vi "EOL CAN_Send_Single_Message.vi"(4 "Retries":i32=2, 6 "Msg Wait Time":u32=100, 7 "Rx Arbitration Id":u32=402522244 format="%.0x", 8 "Error in":errorcluster, 9 "Tx CAN frame":T1={"timestamp"=timestamp(0 s since 1904-01-01), "payload"=[2, 39, 3, 85, 85, 85, 85, 85], "identifier"=402391172, "type"=0, "extended?"=TRUE, "echo?"=FALSE} {"payload" format="%x"; "timestamp" format="%<%.7X\n%x>T"; "type" items=["CAN Data"=0, "CAN Remote"=1, "CAN Bus Error"=2, "CAN 2.0 Data"=8, "CAN FD Data"=16, "CAN FD+BRS Data"=24, "J1939 Data"=192, "Delay"=224, "Log Trigger"=225, "Start Trigger"=226]; "identifier" format="%x"}, 10 "Read Session in":refnum<k21>, 11 "Write Session in":refnum<k21>) -> (0 "Error out":errorcluster, 1 "Rx Message":u8[](array[numeric]) format="%02x", 2 "spreadsheet string":string, 3 "Response Good?":bool, 5 "TxRx Data":string[][](array[string]))   [LabVIEW 2018]
uses:
  <vilib>/xnet/xnet.llb/XNET Frame CAN.ctl
  <vilib>/xnet/xnet.llb/XNET Frame Type CAN.ctl
  <vilib>/xnet/xnet.llb/XNET Write (Frame CAN).vi
  <vilib>/xnet/xnet.llb/XNET Read (Frame CAN).vi
panel:
  # "17FC0084"
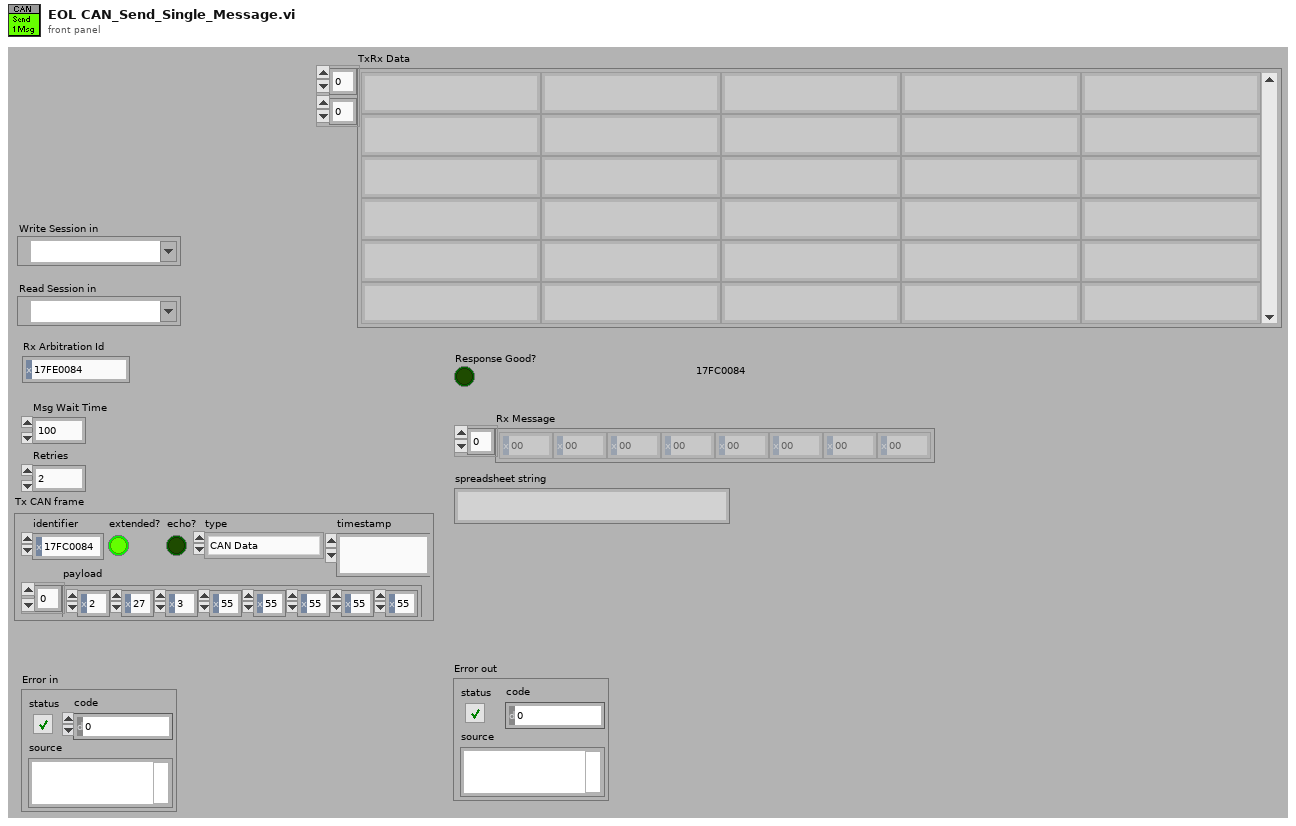
[diagram p1: front panel]
types:
  T1 = typedef "XNET Frame CAN.ctl" = cluster{"timestamp":timestamp, "payload":u8[], "identifier":u32, "type":T2, "extended?":bool, "echo?":bool}
  T2 = typedef "XNET Frame Type CAN.ctl" = u8
  T3 = cluster{"Read Session in":refnum<k21>, "Write Session in":refnum<k21>, "Tx CAN frame":T1, "Rx Arbitration Id":u32, "Retry Counter":i32, "Rx Msg":u8[], "Response Good?":bool, "TxRx Data":string[][], "Message Start Timer":u32, "Message Wait Timer":i32, "Error in":errorcluster}
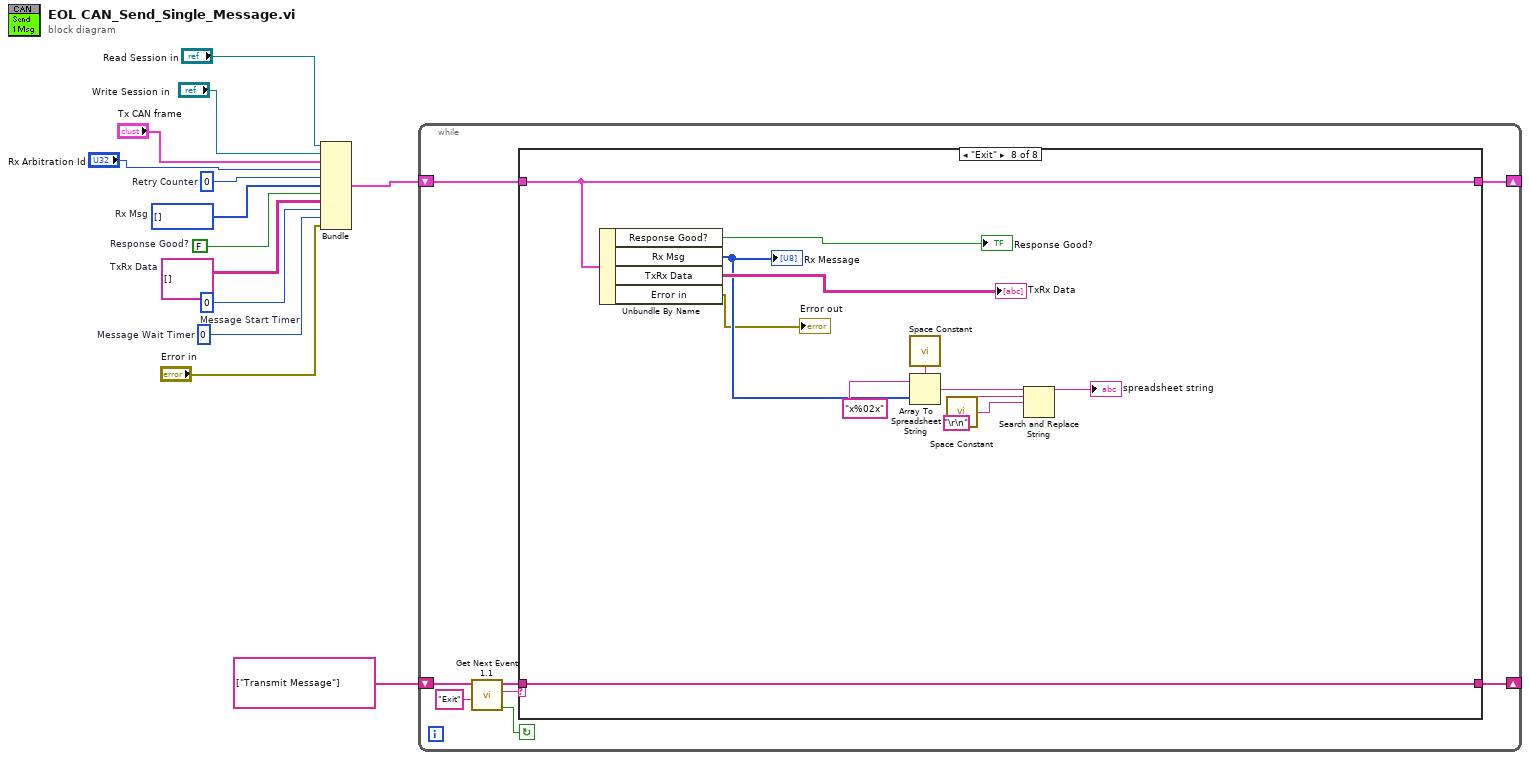
[diagram p0: block diagram]
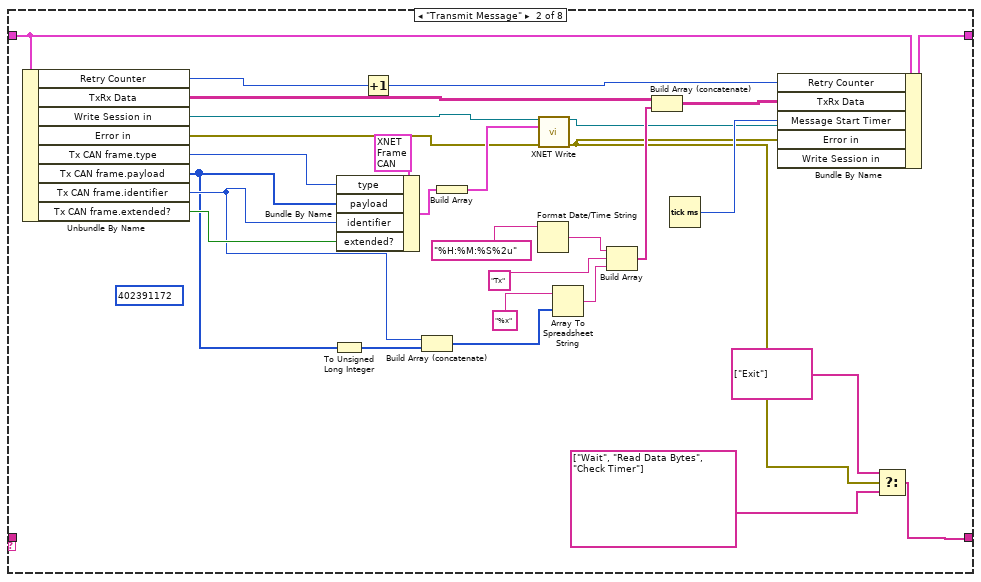
[diagram p3: hidden frame]
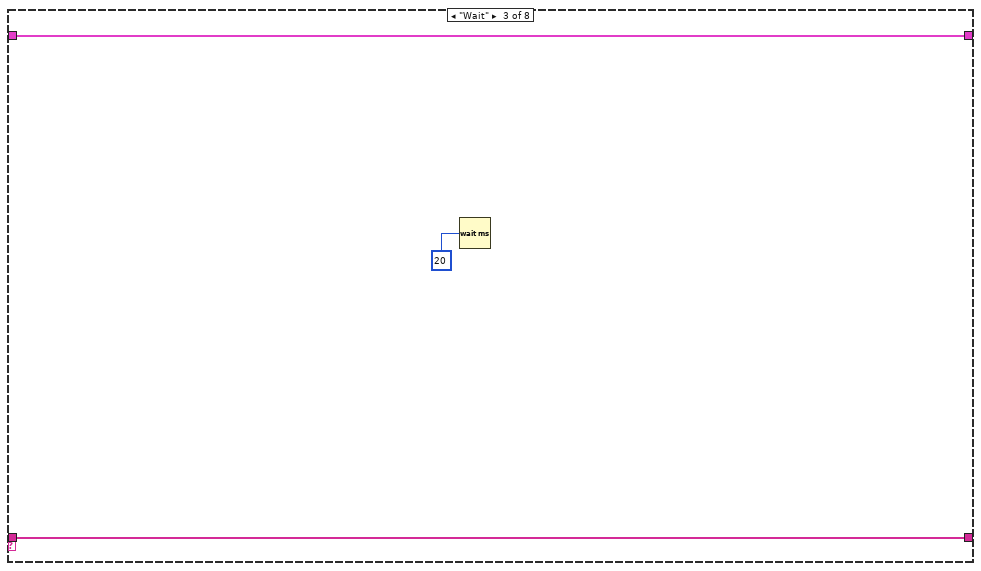
[diagram p4: hidden frame]
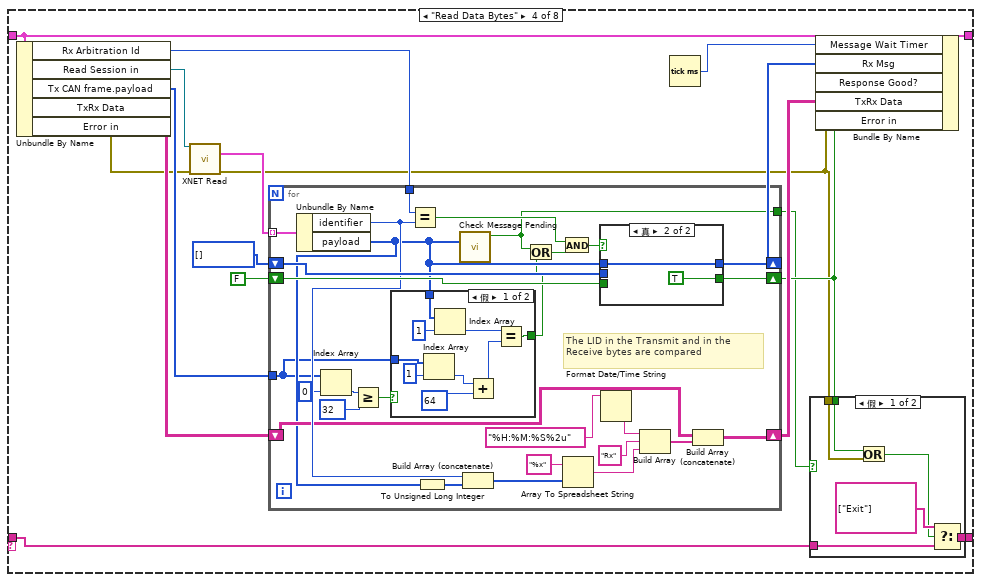
[diagram p5: hidden frame]
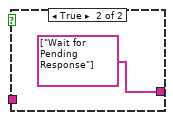
[diagram p6: hidden frame]
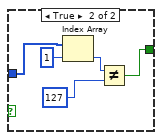
[diagram p7: hidden frame]
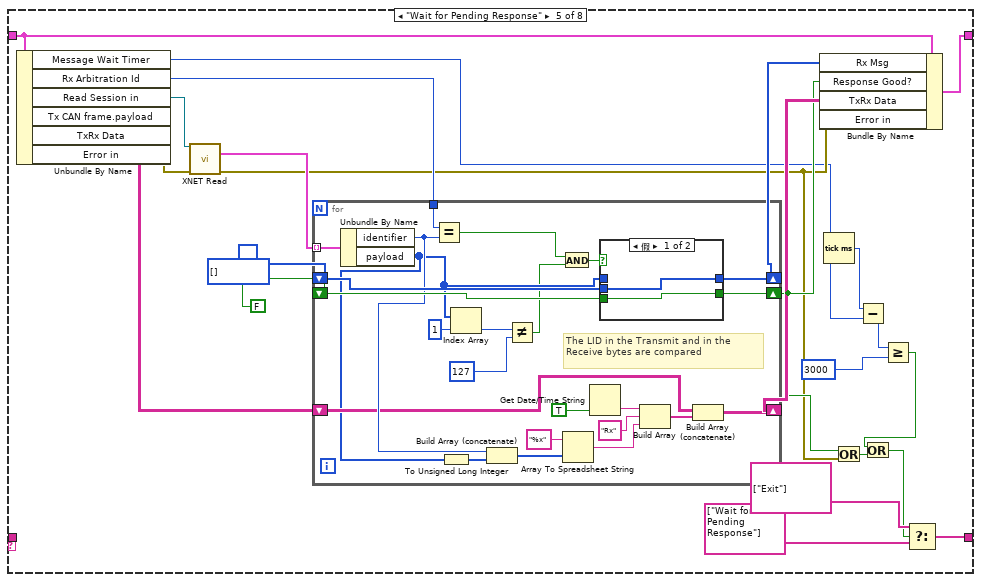
[diagram p9: hidden frame]
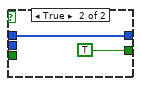
[diagram p10: hidden frame]
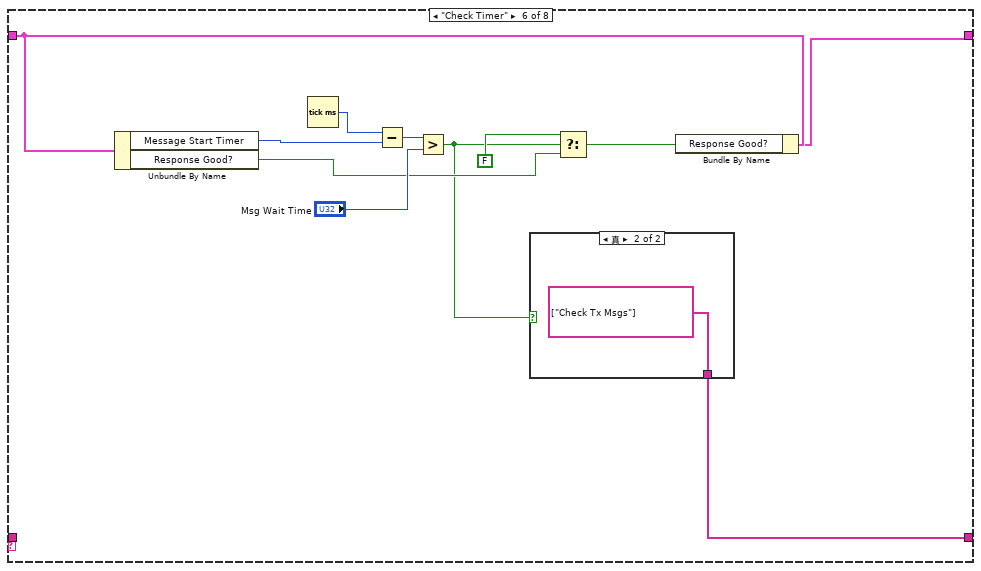
[diagram p11: hidden frame]
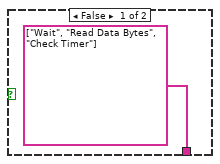
[diagram p12: hidden frame]
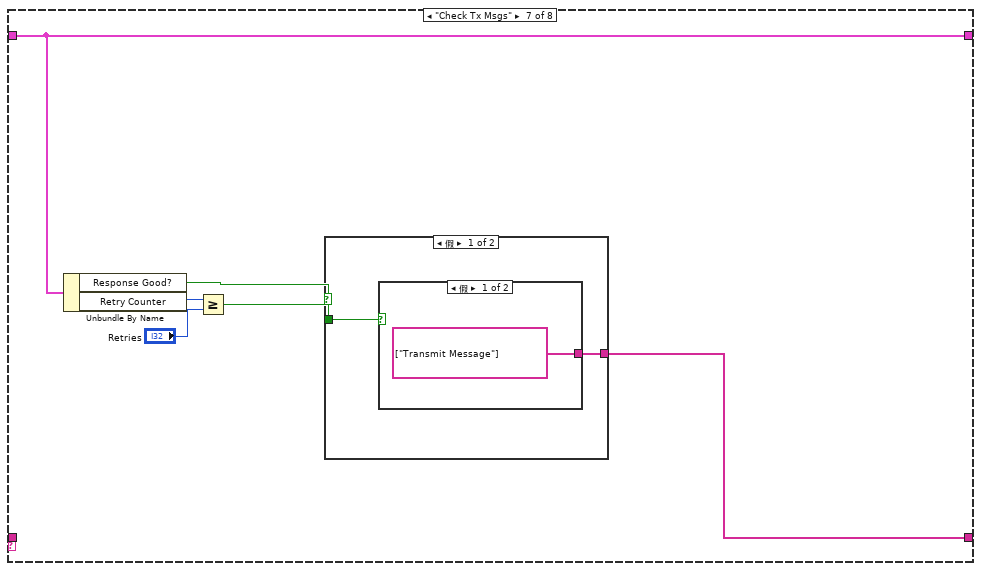
[diagram p13: hidden frame]
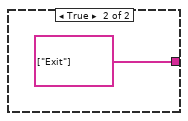
[diagram p14: hidden frame]
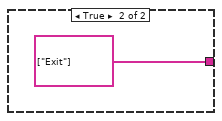
[diagram p15: hidden frame]
diagram:
  w1 = 0  # Message Wait Timer
  w7 = u32 0  # Message Start Timer
  w8 = string[][] []  # TxRx Data
  w9 = FALSE  # Response Good?
  w10 = u8[] []  # Rx Msg
  w12 = 0  # Retry Counter
  n1 = Bundle("Read Session in"="Read Session in", "Write Session in"="Write Session in", "Tx CAN frame"="Tx CAN frame", "Rx Arbitration Id"="Rx Arbitration Id", "Retry Counter"=w12, "Rx Msg"=w10, "Response Good?"=w9, "TxRx Data"=w8, "Message Start Timer"=w7, "Message Wait Timer"=w1, "Error in"="Error in") -> (w11:T3)  [unwired: 1 in]
  n2 = while {
    shift-right: [w18] -> _
    shift-left: string[] ["Transmit Message"] ("event queue out") -> [w17]
    shift-right: [w15] -> _
    shift-left: w11 -> [w16]
    stop <- w21 continue-if-true
    n3 = call "Get Next Event 1.1.vi"("Exit Event"="Exit", "event queue in"=w17) -> ("Condition (Exit:F)"=w21:bool, "next event"=w20:string, "event queue out"=w19:string[])  [unwired: 6 in, 1 out]
    n4 = case shown="\"Exit\"" w20 {
      tunnel: w19 -> [w23 _ w53 w68 _ _ _ w213]
      tunnel: [w23 w32 w53 w67 w145 w178 w193 w213] -> w18
      tunnel: w16 -> [w22 w51 w54 w73 w149 w180 w191 w212]
      tunnel: [w22 w49 w54 w72 w148 w179 w191 w212] -> w15
      frame "Error", Default {
      }
      frame "Transmit Message" {
        (unwired) u32 402391172 ("Tx Arbitration Id")
        n5 = Unbundle By Name(w51) -> ("Retry Counter"=w52:i32, "TxRx Data"=w46:string[][], "Write Session in"=w27:refnum<k21>, "Error in"=w26:errorcluster, "Tx CAN frame.type"=w33:T2, "Tx CAN frame.payload"=w34:u8[], "Tx CAN frame.identifier"=w35:u32, "Tx CAN frame.extended?"=w36:bool)
        n6 = To Unsigned Long Integer(number=w34) -> (unsigned 32bit integer=w45:u32[])
        n7 = Bundle By Name(cluster=T1 {"timestamp"=timestamp(0 s since 1904-01-01), "payload"=[2, 39, 3, 85, 85, 85, 85, 85], "identifier"=402391172, "type"=8, "extended?"=TRUE, "echo?"=FALSE} ("CAN frame"), "type"=w33, "payload"=w34, "identifier"=w35, "extended?"=w36) -> (w39:T1)
        n8 = Increment(x=w52) -> (x+1=w50:i32)
        n9 = Build Array (concatenate)(w35, w45) -> (w41:u32[])
        n10 = Build Array(w39) -> (w37:T1[])
        n11 = Format Date/Time String(time format string (%c)="%H:%M:%S%2u" ("时间格式字符串(%c)")) -> (date/time string=w25:string)  [unwired: 2 in]
        n12 = call-poly <vilib>:"XNET Write.vi"("session in"=w27, "data"=w37, "error in (no error)"=w26) -> ("session out"=w28:refnum<k21>, "error out"=w29:errorcluster)  [unwired: 11 in]
        n13 = Array To Spreadsheet String(array=w41, 3:"%x" ("format string")) -> (spreadsheet string=w43:string)  [unwired: 1 in]
        n14 = Build Array(w25, "Tx" ("format string"), w43) -> (w44:string[])
        n15 = Build Array (concatenate)(w46, w44) -> (w47:string[][])
        n16 = Tick Count (ms)() -> (millisecond timer value=w48:u32)
        n17 = Bundle By Name(cluster=w51, "Retry Counter"=w50, "TxRx Data"=w47, "Message Start Timer"=w48, "Error in"=w29, "Write Session in"=w28) -> (w49:T3)
        n18 = Select(t=string[] ["Exit"], s=w29, f=string[] ["Wait", "Read Data Bytes", "Check Timer"] ("event queue out")) -> (s? t:f=w32:string[])
      }
      frame "Wait" {
        n19 = Wait (ms)(milliseconds to wait=u32 20) -> ()  [unwired: 1 out]
      }
      frame "Read Data Bytes" {
        n20 = Unbundle By Name(w73) -> ("Rx Arbitration Id"=w60:u32, "Read Session in"=w70:refnum<k21>, "Tx CAN frame.payload"=w69:u8[], "TxRx Data"=w66:string[][], "Error in"=w64:errorcluster)
        n21 = call-poly <vilib>:"XNET Read.vi"("session in"=w70, "error in (no error)"=w64) -> ("data"=w61:T1[], "error out"=w58:errorcluster)  [unwired: 10 in, 2 out]
        n22 = for {
          tunnel: w61 -> [w108] mode=indexing
          shift-right: [w107] -> w71
          shift-left: u8[] [] ("Data Array") -> [w106]
          shift-right: [w105] -> w59
          shift-left: FALSE -> [w104]
          tunnel: w69 -> [w86]
          shift-right: [w94] -> w65
          shift-left: w66 -> [w95]
          tunnel: w60 -> [w92]
          tunnel: [w88] -> w57
          # "The LID in the Transmit and in the\nReceive bytes are compared"
          n23 = Unbundle By Name(w108) -> ("identifier"=w100:u32, "payload"=w91:u8[])
          n24 = Index Array(array=w86, index=0) -> (element=w85:u8)
          n25 = Greater Or Equal?(x=w85, y=u8 32) -> (x >= y?=w83:bool)
          n26 = case shown="假" w83 {
            tunnel: w91 -> [w114 _]
            tunnel: [w113 w119] -> w90
            tunnel: w86 -> [w112 w118]
            frame False {
              n27 = Index Array(array=w112, index=1) -> (element=w111:u8)
              n28 = Index Array(array=w114, index=1) -> (element=w117:u8)
              n29 = Add(x=w111, y=u8 64 ("Numeric")) -> (x+y=w116:u8)
              n30 = Equal?(x=w117, y=w116) -> (x = y?=w113:bool)
            }
            frame True {
              n31 = Index Array(array=w118, index=1) -> (element=w120:u8)
              n32 = Not Equal?(x=w120, y=u8 127 ("Numeric")) -> (x != y?=w119:bool)
            }
          }
          n33 = Equal?(x=w92, y=w100) -> (x = y?=w102:bool)
          n34 = To Unsigned Long Integer(number=w91) -> (unsigned 32bit integer=w101:u32[])
          n35 = call "Check Message Pending.vi"("Data Array"=w91) -> ("x .and. y?"=w88:bool)  [unwired: 10 in]
          n36 = Build Array (concatenate)(w100, w101) -> (w93:u32[])
          n37 = Or(x=w88, y=w90) -> (x .or. y?=w89:bool)
          n38 = And(x=w102, y=w89) -> (x .and. y?=w103:bool)
          n39 = Array To Spreadsheet String(array=w93, 3:"%x" ("format string")) -> (spreadsheet string=w97:string)  [unwired: 1 in]
          n40 = case shown="真" w103 {
            tunnel: w91 -> [_ w125]
            tunnel: [w123 w125] -> w107
            tunnel: w106 -> [w123 _]
            tunnel: [w124 TRUE] -> w105
            tunnel: w104 -> [w124 _]
            frame False {
            }
            frame True {
            }
          }
          n41 = Format Date/Time String(time format string (%c)="%H:%M:%S%2u" ("时间格式字符串(%c)")) -> (date/time string=w82:string)  [unwired: 2 in]
          n42 = Build Array(w82, "Rx" ("format string"), w97) -> (w96:string[])
          n43 = Build Array (concatenate)(w95, w96) -> (w94:string[][])
        }
        n44 = Tick Count (ms)() -> (millisecond timer value=w56:u32)
        n45 = case shown="假" w57 {
          tunnel: w68 -> [w79 _]
          tunnel: [w78 string[] ["Wait for Pending Response"] ("t")] -> w67
          tunnel: w59 -> [w76 _]
          tunnel: w58 -> [w74 _]
          frame False {
            n46 = Or(x=w76, y=w74) -> (x .or. y?=w75:bool)
            n47 = Select(t=string[] ["Exit"], s=w75, f=w79) -> (s? t:f=w78:string[])
          }
          frame True {
          }
        }
        n48 = Bundle By Name(cluster=w73, "Message Wait Timer"=w56, "Rx Msg"=w71, "Response Good?"=w59, "TxRx Data"=w65, "Error in"=w58) -> (w72:T3)
      }
      frame "Wait for Pending Response" {
        n49 = Unbundle By Name(w149) -> ("Message Wait Timer"=w131:i32, "Rx Arbitration Id"=w138:u32, "Read Session in"=w146:refnum<k21>, "TxRx Data"=w144:string[][], "Error in"=w142:errorcluster)  [unwired: 1 out]
        n50 = call-poly <vilib>:"XNET Read.vi"("session in"=w146, "error in (no error)"=w142) -> ("data"=w139:T1[], "error out"=w136:errorcluster)  [unwired: 10 in, 2 out]
        n51 = for {
          tunnel: w139 -> [w173] mode=indexing
          shift-right: [w172] -> w147
          shift-left: u8[] [] ("Data Array") -> [w171]
          shift-right: [w170] -> w137
          shift-left: FALSE -> [w169]
          shift-right: [w155] -> w143
          shift-left: w144 -> [w156]
          tunnel: w138 -> [w153]
          # "The LID in the Transmit and in the\nReceive bytes are compared"
          n52 = Unbundle By Name(w173) -> ("identifier"=w163:u32, "payload"=w152:u8[])
          n53 = Equal?(x=w153, y=w163) -> (x = y?=w167:bool)
          n54 = To Unsigned Long Integer(number=w152) -> (unsigned 32bit integer=w164:u32[])
          n55 = Index Array(array=w152, index=1) -> (element=w166:u8)
          n56 = Build Array (concatenate)(w163, w164) -> (w154:u32[])
          n57 = Not Equal?(x=w166, y=u8 127 ("Numeric")) -> (x != y?=w151:bool)
          n58 = And(x=w167, y=w151) -> (x .and. y?=w168:bool)
          n59 = Array To Spreadsheet String(array=w154, 3:"%x" ("format string")) -> (spreadsheet string=w158:string)  [unwired: 1 in]
          n60 = Get Date/Time String(want seconds? (F)=TRUE) -> (time string=w160:string)  [unwired: 2 in, 1 out]
          n61 = case shown="假" w168 {
            tunnel: w152 -> [_ w176]
            tunnel: [w175 w176] -> w172
            tunnel: w171 -> [w175 _]
            tunnel: [w174 TRUE] -> w170
            tunnel: w169 -> [w174 _]
            frame False {
            }
            frame True {
            }
          }
          n62 = Build Array(w160, "Rx" ("format string"), w158) -> (w157:string[])
          n63 = Build Array (concatenate)(w156, w157) -> (w155:string[][])
        }
        n64 = Bundle By Name(cluster=w149, "Rx Msg"=w147, "Response Good?"=w137, "TxRx Data"=w143, "Error in"=w136) -> (w148:T3)
        n65 = Tick Count (ms)() -> (millisecond timer value=w130:u32)
        n66 = Or(x=w137, y=w136) -> (x .or. y?=w133:bool)
        n67 = Subtract(x=w130, y=w131) -> (x-y=w129:u32)
        n68 = Greater Or Equal?(x=w129, y=u32 3000) -> (x >= y?=w128:bool)
        n69 = Or(x=w128, y=w133) -> (x .or. y?=w132:bool)
        n70 = Select(t=string[] ["Exit"], s=w132, f=string[] ["Wait for Pending Response"] ("t")) -> (s? t:f=w145:string[])
      }
      frame "Check Timer" {
        n71 = Unbundle By Name(w180) -> ("Message Start Timer"=w187:u32, "Response Good?"=w183:bool)
        n72 = Tick Count (ms)() -> (millisecond timer value=w188:u32)
        n73 = Subtract(x=w188, y=w187) -> (x-y=w186:u32)
        n74 = Greater?(x=w186, y="Msg Wait Time") -> (0:w181:bool)
        n75 = case shown="真" w181 {
          tunnel: [string[] ["Wait", "Read Data Bytes", "Check Timer"] ("event queue out") string[] ["Check Tx Msgs"] ("Events to Insert")] -> w178
          frame False {
          }
          frame True {
          }
        }
        n76 = Select(t=FALSE, s=w181, f=w183) -> (s? t:f=w182:bool)
        n77 = Bundle By Name(cluster=w180, "Response Good?"=w182) -> (w179:T3)
      }
      frame "Check Tx Msgs" {
        n78 = Unbundle By Name(w191) -> ("Response Good?"=w194:bool, "Retry Counter"=w195:i32)
        n79 = Greater Or Equal?(x=w195, y="Retries") -> (x >= y?=w192:bool)
        n80 = case shown="假" w194 {
          tunnel: [w197 string[] ["Exit"] ("event queue out")] -> w193
          tunnel: w192 -> [w198 _]
          frame False {
            n81 = case shown="假" w198 {
              tunnel: [string[] ["Transmit Message"] ("f") string[] ["Exit"] ("event queue out")] -> w197
              frame False {
              }
              frame True {
              }
            }
          }
          frame True {
          }
        }
      }
      frame "Exit" {
        n82 = Unbundle By Name(w212) -> ("Response Good?"=→"Response Good?":bool, "Rx Msg"=w204:u8[], "TxRx Data"=→"TxRx Data":string[][], "Error in"=→"Error out":errorcluster)
        "Rx Message" <- w204
        n83 = call <vilib>:"Space Constant.vi"() -> ("String"=w206:string)
        n84 = Array To Spreadsheet String(delimiter (Tab)=w206, array=w204, 3:"x%02x" ("format string")) -> (spreadsheet string=w205:string)
        n85 = call <vilib>:"Space Constant.vi"() -> ("String"=w208:string)
        n86 = Search and Replace String(input string=w205, search string="\r\n", replace string=w208) -> (result string=→"spreadsheet string":string)  [unwired: 5 in, 3 out]
      }
    }
  }
